vi "Request Synchronous Data (Variant).vi"(6 "Ignore Past Updates? (F)":bool, 7 "Timeout In ms (-1)":i32=-1, 8 "error in (no error)":errorcluster, 9 "Type":variant, 10 "Datum Name":string, 11 "IModel In":refnum<class "IModel.lvclass">) -> (0 "error out":errorcluster, 1 "timed out?":bool, 2 "Data":variant, 4 "Publication Time":timestamp)   [LabVIEW 2015, in "IModel.lvlib" / "IModel.lvclass"]
doc: "<License>\nCopyright © 2017 Composed Systems, LLC | All rights reserved\nwww.composed.io\n\nAuthor: Ethan Stern <ethan.stern@composed.io>\n\nThis software is provided \"AS IS\" WITHOUT WARRANTIES, either express or implied, AND IS FOR EDUCATIONAL PURPOSES ONLY.\n</License>"
uses:
  IModel.lvclass
  <vilib>/ActorFramework/Actor/Actor.lvclass/Actor.ctl
  <vilib>/ActorFramework/Message Enqueuer/Message Enqueuer.lvclass/Message Enqueuer.ctl
  IModel.lvclass/IModel.ctl
  SubscriptionPolicy/OneShotSubscription/OneShotSubscription.lvclass/OneShotSubscription.ctl
  AbstractMessages/PreAddressedMsg/PreAddressedMsg.lvclass/PreAddressedMsg.ctl
  IMediator/IMediator Messages/Subscribe Msg/Subscribe Msg.lvclass/Subscribe Msg.ctl
  <vilib>/ActorFramework/Message Enqueuer/Init from Existing Queue.vi
  <vilib>/ActorFramework/Message Enqueuer/Enqueue.vi
  AbstractMessages/PreAddressedMsg/Read Return Address.vi
  <vilib>/ActorFramework/Message Priority Queue/Priority Enqueue.vi
  <vilib>/ActorFramework/Message Enqueuer/Message Enqueuer.lvclass
  SubscriptionPolicy/OneShotSubscription/OneShotSubscription.lvclass
  Transport/QueueTransport/QueueTransport.lvclass
  IMediator/SubscriptionRequest/SubscriptionRequest.lvclass
  IMediator/ISubscriptionPolicy/ISubscriptionPolicy.lvclass
  <vilib>/ActorFramework/Actor/Actor.lvclass
  IMediator/IMediator Messages/Subscribe Msg/Subscribe Msg.lvclass
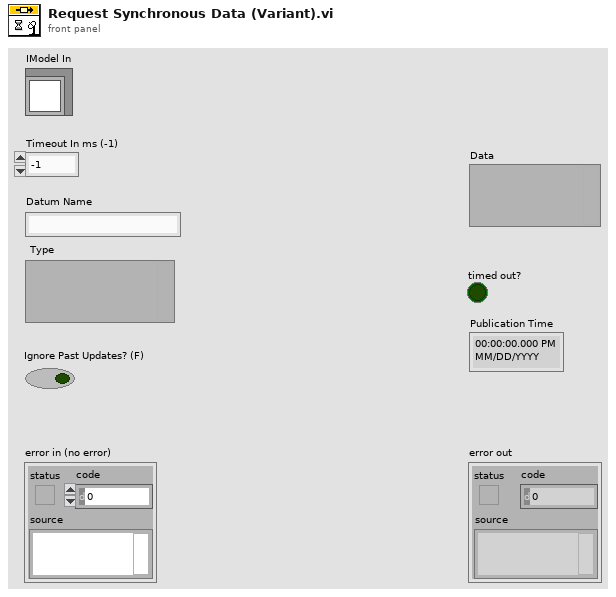
[diagram p1: front panel]
types:
  T1 = typedef "IMediator.lvlib/ISubscriptionPolicy.lvclass/ISubscriptionPolicy Reference.ctl" = refnum<data-value>
  T2 = cluster{"Data":variant, "Publication Time":timestamp}
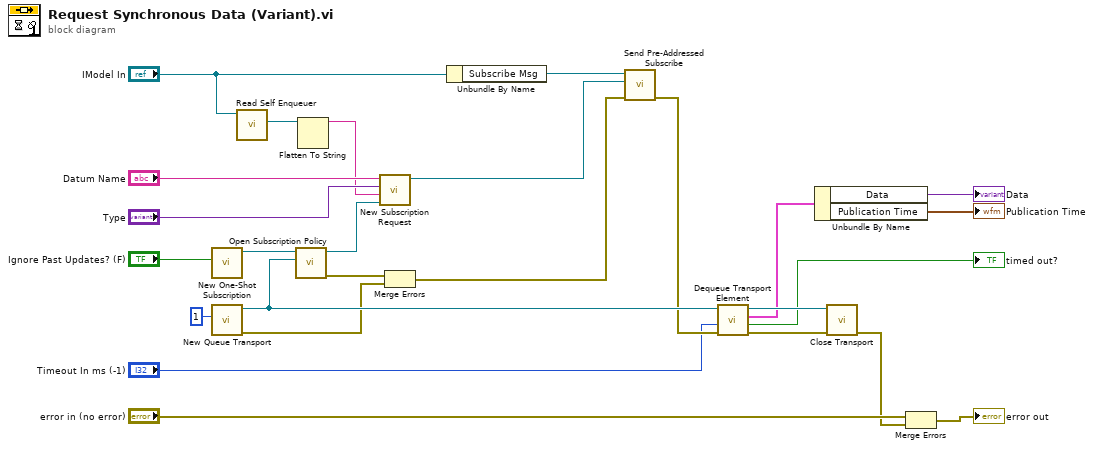
[diagram p0: block diagram]
diagram:
  n1 = call "New One-Shot Subscription.vi"("Ignore Past Updates? (F)"="Ignore Past Updates? (F)") -> ("OneShotSubscription Out"=w19:refnum<class "OneShotSubscription.lvclass">)  [unwired: 10 in]
  n2 = call "New Queue Transport.vi"("Max Queue Size (-1)"=1 ("Max Queue Size (-1, unlimited)")) -> ("error out"=w10:errorcluster, "QueueTransport Out"=w12:refnum<class "QueueTransport.lvclass">)  [unwired: 9 in]
  n3 = call <vilib>:"Read Self Enqueuer.vi"("Actor"="IModel In") -> ("Self Enqueuer"=w21:refnum<class "Message Enqueuer.lvclass">)  [unwired: 10 in]
  n4 = call "Open Subscription Policy.vi"("Transport"=w12, "SubscriptionPolicy"=w19) -> ("error out"=w13:errorcluster, "Subscription Policy"=w22:T1)  [unwired: 8 in]
  n5 = Flatten To String(anything=w21) -> (data string=w17:string)  [unwired: 3 in, 2 out]
  n6 = call "New Subscription Request.vi"("Subscription Policy"=w22, "Unique Subscriber ID"=w17, "Type"="Type", "Datum Name"="Datum Name") -> ("SubscriptionRequest"=w14:refnum<class "SubscriptionRequest.lvclass">)  [unwired: 7 in]
  n7 = Merge Errors(w13, w10) -> (w11:errorcluster)
  n8 = Unbundle By Name("IModel In") -> ("Subscribe Msg"=w15:refnum<class "Subscribe Msg.lvclass">)
  n9 = call "Send Pre-Addressed Subscribe.vi"("error in (no error)"=w11, "Subscription Request"=w14, "Subscribe Msg"=w15) -> ("error out"=w9:errorcluster)  [unwired: 8 in]
  n10 = call "Dequeue Transport Element.vi"("error in (no error)"=w9, "Timeout In ms (-1)"="Timeout In ms (-1)", "QueueTransport in"=w12) -> ("error out"=w6:errorcluster, "timed out?"=→"timed out?":bool, "Element"=w3:T2, "QueueTransport out"=w26:refnum<class "QueueTransport.lvclass">)  [unwired: 5 in]
  n11 = Unbundle By Name(w3) -> ("Data"=→"Data":variant, "Publication Time"=→"Publication Time":timestamp)
  n12 = call-dynamic "Close Transport.vi"("error in (no error)"=w6, "QueueTransport in"=w26) -> ("error out"=w4:errorcluster)  [unwired: 9 in]
  n13 = Merge Errors("error in (no error)", w4) -> (→"error out":errorcluster)
